vi "PCO_FreeBuffer.vi"(8 "error in (no error)":errorcluster, 10 "sBufNr":i16, 11 "Handle":u64) -> (0 "error out":errorcluster, 3 "Handle Out":u64, 5 "return type":u32 format="%x")   [LabVIEW 2011]
uses:
  SC2_Cam64.dll
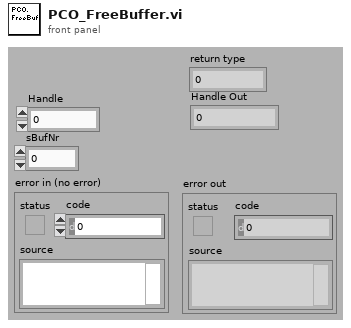
[diagram p1: front panel]
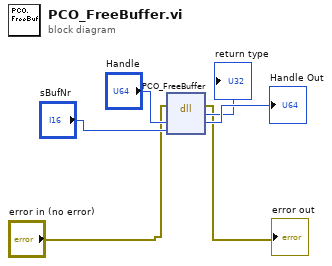
[diagram p0: block diagram]
diagram:
  n1 = dll-call lib="C:/Program Files/colibri/Drivers/PCO.Camera/SC2_Cam*.*" fn="PCO_FreeBuffer"(error in="error in (no error)", "Handle"="Handle", "sBufNr"="sBufNr") -> (error out=→"error out":errorcluster, "return type"=→"return type":u32, "Handle"=→"Handle Out":u64)  [unwired: 3 in, 1 out]
